vi "Get folder file list with subs.vi"() -> ()   [LabVIEW 2013]
uses:
  <vilib>/Utility/file.llb/Write To Spreadsheet File (string).vi
panel:
  out "File paths and mod date":string[][](array[string])
  in  "Folder Path":path
  in  "pattern":string
  out "error out":errorcluster
  in  "error in (no error)":errorcluster
  out "All Folders":path[](array[path])
  out "Number of Files":i32
  out "All Files in Dir":path[](array[path])
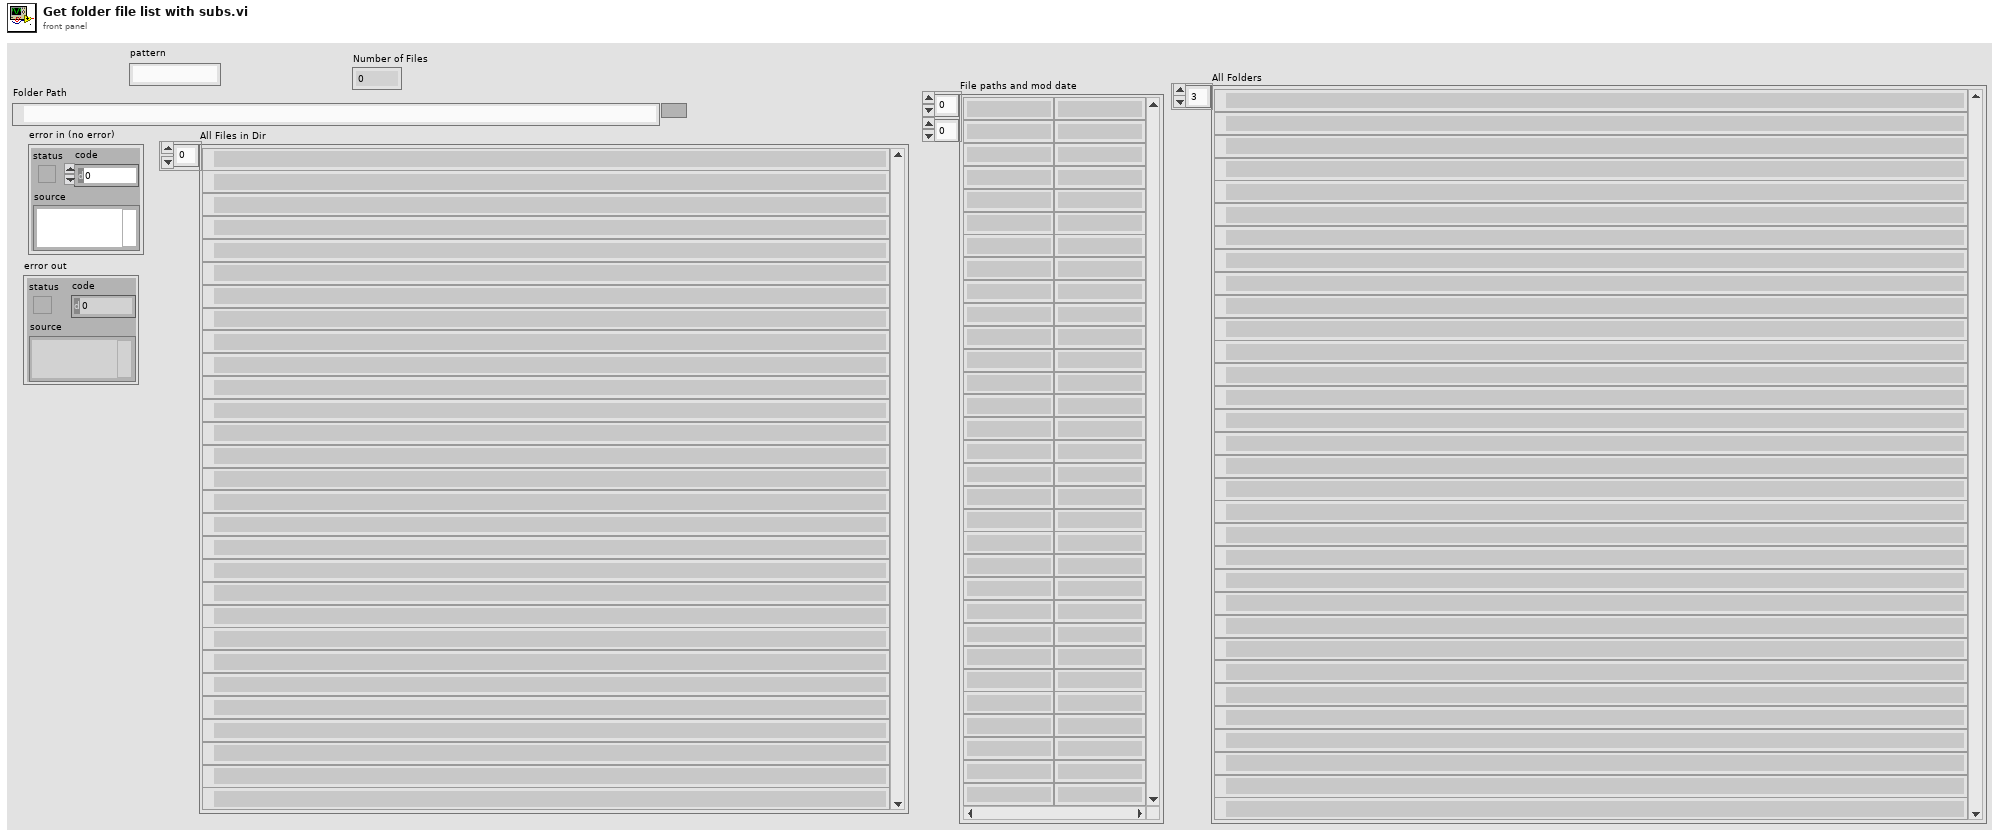
[diagram p1: front panel]
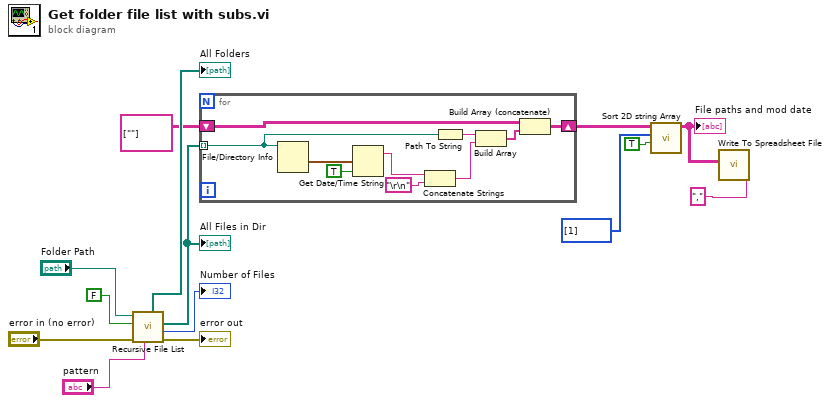
[diagram p0: block diagram]
diagram:
  n1 = call <vilib>:"Recursive File List.vi"("pattern"="pattern", "error in (no error)"="error in (no error)", "Treat LLBs as Folders?"=FALSE, "Folder Path"="Folder Path") -> ("error out"=→"error out":errorcluster, "Number of Files"=→"Number of Files":i32, "All Files in Dir"=w7:path[], "All Folders"=→"All Folders":path[])  [unwired: 3 in, 1 out]
  "All Files in Dir" <- w7
  n2 = for {
    tunnel: w7 -> [w22] mode=indexing
    shift-right: [w15] -> w5
    shift-left: string[][] [[""]] -> [w19]
    n3 = File/Directory Info(path=w22) -> (last mod=w24:timestamp)  [unwired: 1 in, 6 out]
    n4 = Get Date/Time String(seconds (now)=w24, want seconds? (F)=TRUE) -> (date string=w21:string)  [unwired: 1 in, 1 out]
    n5 = Concatenate Strings(w21, "\r\n") -> (w17:string)
    n6 = Path To String(path=w22) -> (string=w18:string)
    n7 = Build Array(w18, w17) -> (w16:string[])
    n8 = Build Array (concatenate)(w19, w16) -> (w15:string[][])
  }
  n9 = call "Sort 2D string Array.vi"("Descending (F)"=TRUE, "Priority Columns (0)"=i32[] [1], "Unsorted Array"=w5) -> ("Sorted array"=w4:string[][])  [unwired: 6 in, 2 out]
  "File paths and mod date" <- w4
  n10 = call-poly <vilib>:"Write To Spreadsheet File.vi"("delimiter (\\t)"="," ("delimiter (\\t)"), "2D data"=w4) -> ()  [unwired: 6 in, 1 out]
